vi "Read Time Stamp.vi"(8 "error in (no error)":errorcluster, 11 "Timestamp Result in":refnum<class "Timestamp Result.lvclass">) -> (0 "error out":errorcluster, 2 "Time Stamp":timestamp, 3 "Timestamp Result out":refnum<class "Timestamp Result.lvclass">)   [LabVIEW 2015, in "Timestamp Result.lvclass"]
uses:
  Timestamp Result.lvclass
  Timestamp Result.lvclass/Timestamp Result.ctl
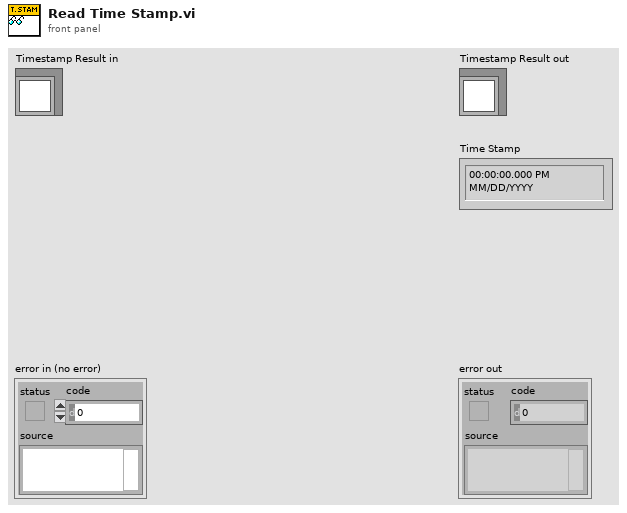
[diagram p1: front panel]
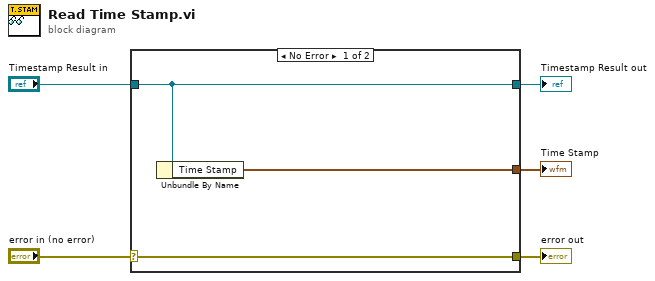
[diagram p0: block diagram]
diagram:
  n1 = case shown="No Error" "error in (no error)" {
    selector: "error in (no error)" -> [w8 w9]
    tunnel: [w8 w9] -> w4
    tunnel: [w7 w10] -> w2
    tunnel: "Timestamp Result in" -> [w7 w10]
    tunnel: [w6 _] -> w1
    frame No Error {
      n2 = Unbundle By Name(w7) -> ("Time Stamp"=w6:timestamp)
    }
    frame Error {
    }
  }
  "error out" <- w4
  "Timestamp Result out" <- w2
  "Time Stamp" <- w1
